vi "Data Item Test.vi"() -> ()   [LabVIEW 2018]
uses:
  Failure Information.ctl
  Log Record.ctl
  Logger/Internal Log Levels.ctl
  Filters/Aggregation Method.ctl
  40037e18-95a9-4cb9-9ddf-d3c11cbaea1d.vi
  40037e18-95a9-4cb9-9ddf-d3c11cbaea1d.vi/a153a250-4fb8-4a99-bb5b-6ccb57f1f631.vi
  40037e18-95a9-4cb9-9ddf-d3c11cbaea1d.vi/a153a250-4fb8-4a99-bb5b-6ccb57f1f631.vi/28727e37-b0d9-407c-a479-ab0b7779cd69.vi
  Filters/Data Item/Data Item.lvclass
  C:/Users/Colin/Documents/software_projects/glog/Logging/Filters/Filter/Filter.lvclass
  Handlers/File Handler/File Handler.lvclass
  C:/Users/Colin/Documents/software_projects/glog/Logging/Handlers/Formatting Handler/Formatting Handler.lvclass
  Filters/Data Item/New (Element).vi
  Filters/Data Item/New (Array).vi
  Registry/Log.vi
  Logging.lvlib
panel:
  out "failures info":T1[](array[typedef]) {"Log Record"."timestamp" format="%<%x %.3X>T"}
  out "error out":errorcluster
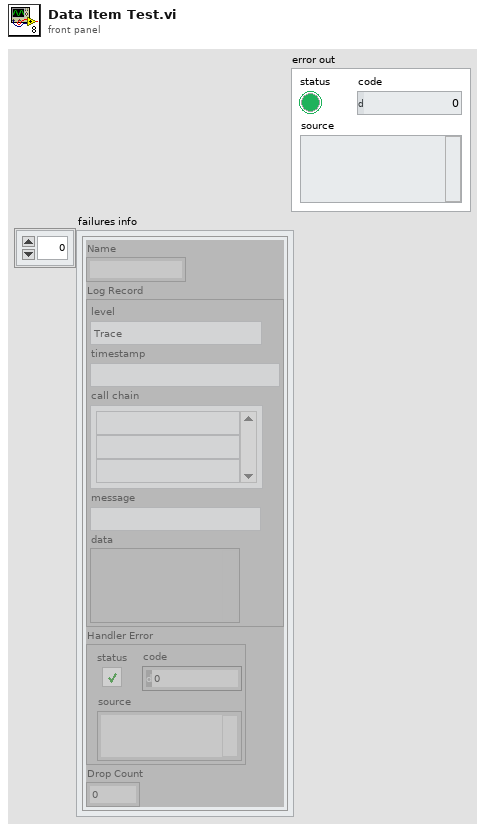
[diagram p1: front panel]
types:
  T1 = typedef "Logging.lvlib/Failure Information.ctl" = cluster{"Name":string, "Log Record":T2, "Handler Error":errorcluster, "Drop Count":u32}
  T2 = typedef "Logging.lvlib/Log Record.ctl" = cluster{"level":T3, "timestamp":timestamp, "call chain":string[], "message":string, "data":variant}
  T3 = typedef "Logging.lvlib/Internal Log Levels.ctl" = enum16{"Trace", "Debug", "Info", "Warning", "Error", "Critical", "Internal"}
  T4 = typedef "Logging.lvlib/Aggregation Method.ctl" = enum16{"Any", "Only", "All", "None"}
  T5 = cluster{"Iteration":i32, "CPU ID":string, "Machine Name":string, "PID":string}
  T6 = cluster{"Iteration":i32, "CPU ID":string, "Machine Name":string}
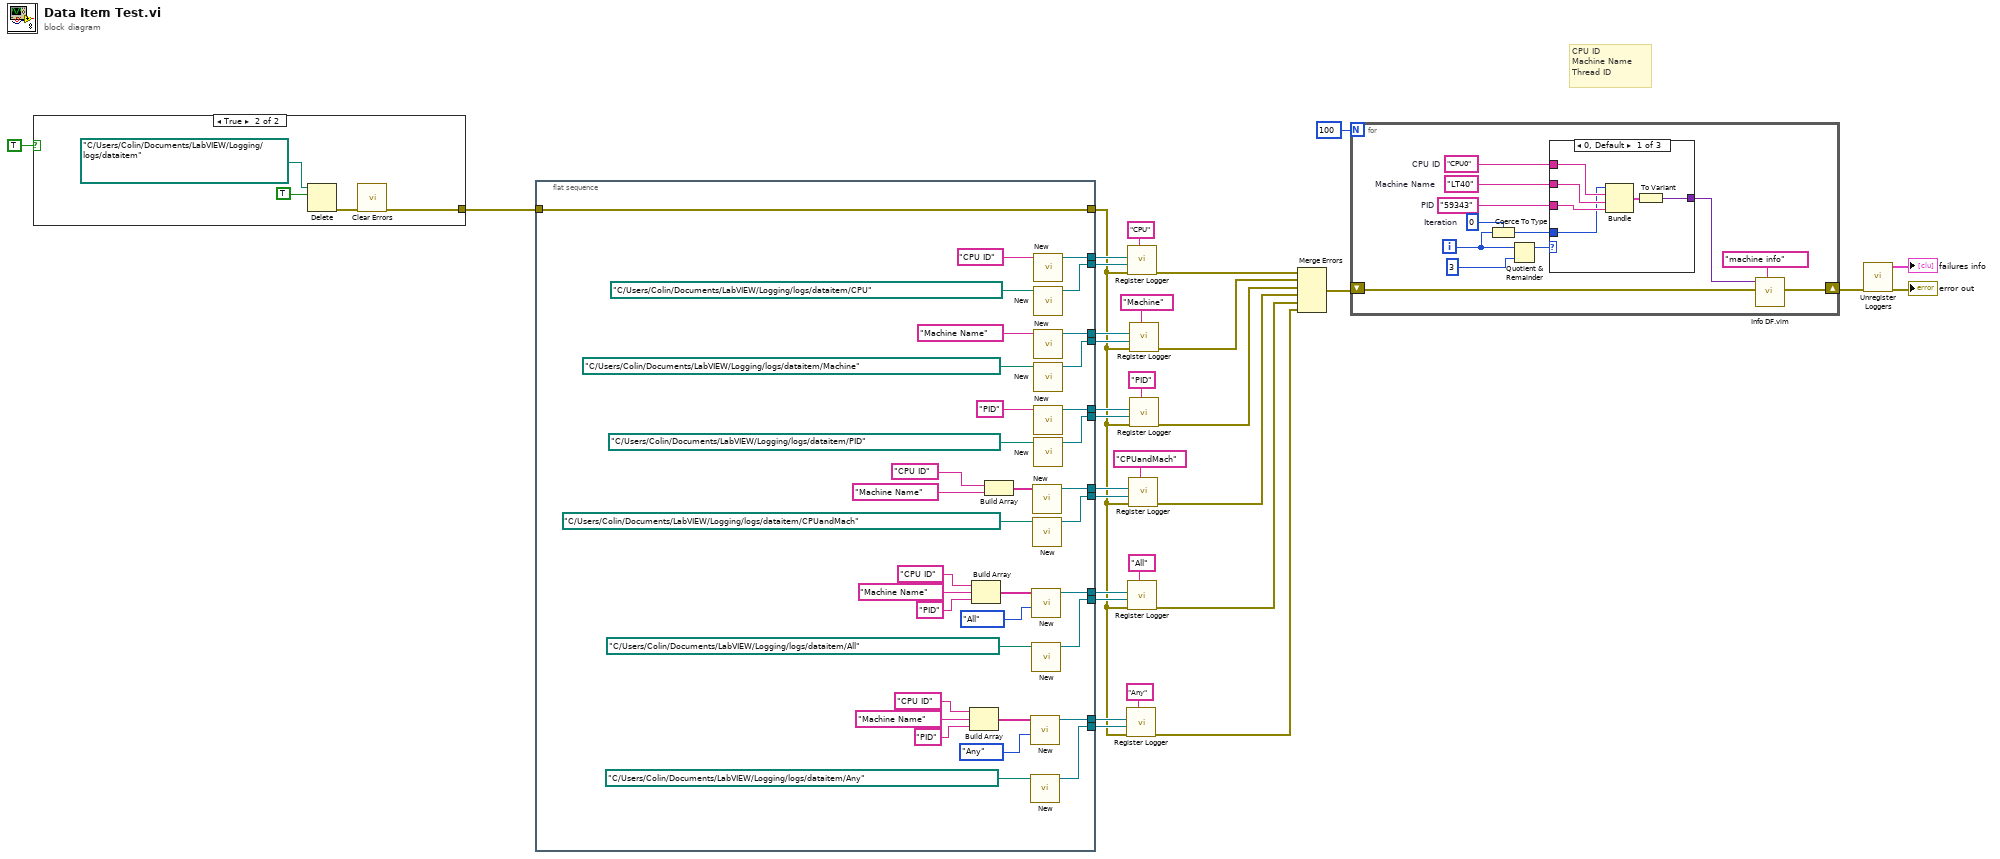
[diagram p0: block diagram]
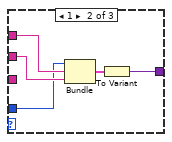
[diagram p2: hidden frame]
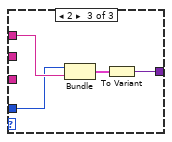
[diagram p3: hidden frame]
diagram:
  # "CPU ID\nMachine Name\nThread ID"
  n1 = case shown="True" TRUE {
    tunnel: [_ w33] -> w21
    frame False {
    }
    frame True {
      n2 = Delete(path (use dialog)=path "C:/Users/Colin/Documents/LabVIEW/Logging/logs/dataitem" ("log directory (<app dir>/logs)"), entire hierarchy (F)=TRUE) -> (error out=w35:errorcluster)  [unwired: 3 in, 2 out]
      n3 = call <vilib>:"Clear Errors.vi"("error in (no error)"=w35) -> ("error out"=w33:errorcluster)  [unwired: 5 in, 1 out]
    }
  }
  n4 = flat-sequence {
    tunnel: [w71] -> w32
    tunnel: [w69] -> w31
    tunnel: [w68] -> w30
    tunnel: [w66] -> w29
    tunnel: w21 -> [w63]
    tunnel: [w63] -> w4
    tunnel: [w59] -> w18
    tunnel: [w61] -> w19
    tunnel: [w58] -> w16
    tunnel: [w57] -> w15
    tunnel: [w53] -> w10
    tunnel: [w54] -> w11
    tunnel: [w48] -> w7
    tunnel: [w47] -> w6
    frame #0 {
      n5 = Build Array("CPU ID" ("regex string"), "Machine Name" ("regex string"), "PID" ("regex string")) -> (w39:string[])
      n6 = Build Array("CPU ID" ("regex string"), "Machine Name" ("regex string"), "PID" ("regex string")) -> (w49:string[])
      n7 = Build Array("CPU ID" ("regex string"), "Machine Name" ("regex string")) -> (w43:string[])
      n8 = call-poly "New.vi"("aggregation method (all)"=Aggregation_Method."Any", "data item names"=w39) -> ("data item out"=w47:refnum<class "Data Item.lvclass">)  [unwired: 8 in, 1 out]
      n9 = call "New.vi"("log directory (<app dir>/logs)"=path "C:/Users/Colin/Documents/LabVIEW/Logging/logs/dataitem/Any") -> ("file handler"=w48:refnum<class "File Handler.lvclass">)  [unwired: 10 in]
      n10 = call-poly "New.vi"("aggregation method (all)"=Aggregation_Method."All", "data item names"=w49) -> ("data item out"=w54:refnum<class "Data Item.lvclass">)  [unwired: 8 in, 1 out]
      n11 = call "New.vi"("log directory (<app dir>/logs)"=path "C:/Users/Colin/Documents/LabVIEW/Logging/logs/dataitem/All") -> ("file handler"=w53:refnum<class "File Handler.lvclass">)  [unwired: 10 in]
      n12 = call-poly "New.vi"("data item names"=w43) -> ("data item out"=w57:refnum<class "Data Item.lvclass">)  [unwired: 9 in, 1 out]
      n13 = call "New.vi"("log directory (<app dir>/logs)"=path "C:/Users/Colin/Documents/LabVIEW/Logging/logs/dataitem/CPUandMach") -> ("file handler"=w58:refnum<class "File Handler.lvclass">)  [unwired: 10 in]
      n14 = call-poly "New.vi"("data item name"="CPU ID" ("regex string")) -> ("data item out"=w71:refnum<class "Data Item.lvclass">)  [unwired: 9 in, 1 out]
      n15 = call "New.vi"("log directory (<app dir>/logs)"=path "C:/Users/Colin/Documents/LabVIEW/Logging/logs/dataitem/CPU") -> ("file handler"=w69:refnum<class "File Handler.lvclass">)  [unwired: 10 in]
      n16 = call-poly "New.vi"("data item name"="Machine Name" ("regex string")) -> ("data item out"=w66:refnum<class "Data Item.lvclass">)  [unwired: 9 in, 1 out]
      n17 = call "New.vi"("log directory (<app dir>/logs)"=path "C:/Users/Colin/Documents/LabVIEW/Logging/logs/dataitem/Machine") -> ("file handler"=w68:refnum<class "File Handler.lvclass">)  [unwired: 10 in]
      n18 = call-poly "New.vi"("data item name"="PID" ("regex string")) -> ("data item out"=w61:refnum<class "Data Item.lvclass">)  [unwired: 9 in, 1 out]
      n19 = call "New.vi"("log directory (<app dir>/logs)"=path "C:/Users/Colin/Documents/LabVIEW/Logging/logs/dataitem/PID") -> ("file handler"=w59:refnum<class "File Handler.lvclass">)  [unwired: 10 in]
    }
  }
  n20 = call "Register Logger.vi"("name (\"Default\")"="Any" ("name (\"Default\")"), "error in (no error)"=w4, "log handler (file handler)"=w7, "log filter (none)"=w6) -> ("error out"=w5:errorcluster)  [unwired: 7 in]
  n21 = call "Register Logger.vi"("name (\"Default\")"="CPU" ("name (\"Default\")"), "error in (no error)"=w4, "log handler (file handler)"=w31, "log filter (none)"=w32) -> ("error out"=w27:errorcluster)  [unwired: 7 in]
  n22 = call "Register Logger.vi"("name (\"Default\")"="All" ("name (\"Default\")"), "error in (no error)"=w4, "log handler (file handler)"=w10, "log filter (none)"=w11) -> ("error out"=w12:errorcluster)  [unwired: 7 in]
  n23 = call "Register Logger.vi"("name (\"Default\")"="CPUandMach" ("name (\"Default\")"), "error in (no error)"=w4, "log handler (file handler)"=w16, "log filter (none)"=w15) -> ("error out"=w14:errorcluster)  [unwired: 7 in]
  n24 = call "Register Logger.vi"("name (\"Default\")"="Machine" ("name (\"Default\")"), "error in (no error)"=w4, "log handler (file handler)"=w30, "log filter (none)"=w29) -> ("error out"=w28:errorcluster)  [unwired: 7 in]
  n25 = call "Register Logger.vi"("name (\"Default\")"="PID" ("name (\"Default\")"), "error in (no error)"=w4, "log handler (file handler)"=w18, "log filter (none)"=w19) -> ("error out"=w20:errorcluster)  [unwired: 7 in]
  n26 = Merge Errors(w27, w28, w20, w14, w12, w5) -> (w24:errorcluster)
  n27 = for {
    N: 100 -> [_]
    shift-right: [w82] -> w2
    shift-left: w24 -> [w83]
    i -> [w74]
    w73 = 0  # Iteration
    w76 = "59343"  # PID
    w77 = "LT40"  # Machine Name
    w78 = "CPU0"  # CPU ID
    n28 = Coerce To Type(0:w74, 1:w73) -> (2:w72:i32)
    n29 = Quotient & Remainder(x=w74, y=3) -> (x-y*floor(x/y)=w80:i32)  [unwired: 1 out]
    n30 = case shown="0, Default" w80 {
      tunnel: w78 -> [w89 w93 w97]
      tunnel: w77 -> [w88 w92 _]
      tunnel: w76 -> [w87 _ _]
      tunnel: [w85 w91 w96] -> w75
      tunnel: w72 -> [w84 w90 w95]
      frame 0, Default {
        n31 = Bundle("Iteration"=w84, "CPU ID"=w89, "Machine Name"=w88, "PID"=w87) -> (w86:T5)  [unwired: 1 in]
        n32 = To Variant(anything=w86) -> (Variant=w85:variant)
      }
      frame 1 {
        n33 = Bundle("Iteration"=w90, "CPU ID"=w93, "Machine Name"=w92) -> (w94:T6)  [unwired: 1 in]
        n34 = To Variant(anything=w94) -> (Variant=w91:variant)
      }
      frame 2 {
        n35 = Bundle("Iteration"=w95, "CPU ID"=w97) -> (w98:cluster{"Iteration":i32, "CPU ID":string})  [unwired: 1 in]
        n36 = To Variant(anything=w98) -> (Variant=w96:variant)
      }
    }
    n37 = call "Info DF.vim"("message"="machine info", "dataflow in"=w83, "data (null)"=w75) -> ("dataflow out"=w82:errorcluster)  [unwired: 8 in]
  }
  n38 = call "Unregister Loggers.vi"("error in (no error)"=w2) -> ("error out"=→"error out":errorcluster, "failures info"=→"failures info":T1[])  [unwired: 9 in]
